vi "Load.vi"(8 "error in (no error)":errorcluster, 11 "Proto in":refnum<class "Proto.lvclass">) -> (0 "error out":errorcluster, 2 "Load":u64, 3 "Proto out":refnum<class "Proto.lvclass">)   [LabVIEW 2021, in "Proto.lvclass"]
uses:
  Proto.lvclass
  Proto.lvclass/Proto.ctl
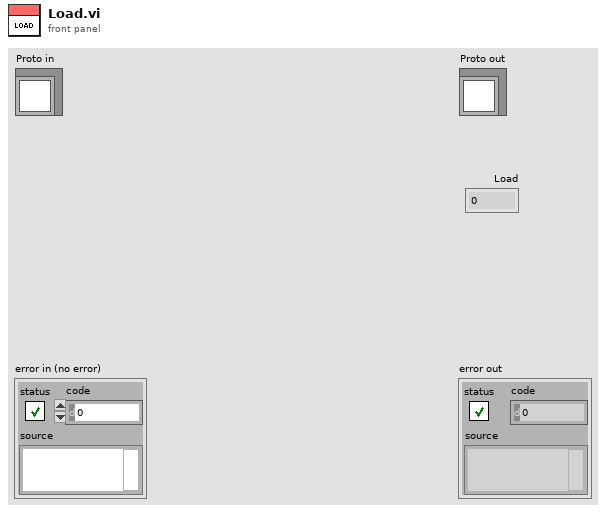
[diagram p1: front panel]
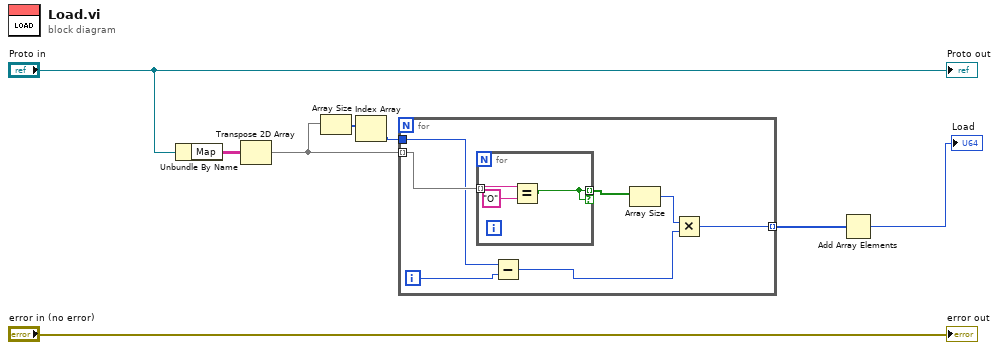
[diagram p0: block diagram]
diagram:
  n1 = Unbundle By Name("Proto in") -> ("Map"=w6:string[][])
  n2 = Transpose 2D Array(2D array=w6) -> (transposed array=w3:string[][])
  n3 = Array Size(array=w3) -> (size(s)=w2:i32[])
  n4 = Index Array(array=w2) -> (element=w1:i32)  [unwired: 1 in]
  n5 = for {
    tunnel: w3 -> [w12] mode=indexing
    tunnel: [w13] -> w4 mode=indexing
    tunnel: w1 -> [w11]
    i -> [w10]
    n6 = for {
      tunnel: w12 -> [w18] mode=indexing
      tunnel: [w16] -> w15 mode=indexing if=w16
      n7 = Equal?(x=w18, y="O") -> (x = y?=w16:bool)
    }
    n8 = Subtract(x=w11, y=w10) -> (x-y=w9:i32)
    n9 = Array Size(array=w15) -> (size(s)=w14:i32)
    n10 = Multiply(x=w14, y=w9) -> (x*y=w13:i32)
  }
  n11 = Add Array Elements(numeric array=w4) -> (sum=→"Load":i32)
  "error out" <- "error in (no error)"
  "Proto out" <- "Proto in"
